vi "OpenConfigFile.vi"(8 "error in (no error)":errorcluster, 10 "ms timeout (2000)":i32=2000, 11 "configuration file path":path) -> (0 "error out":errorcluster, 2 "timeout":bool, 3 "refnum":T1)   [LabVIEW 2020, in "ViewableActor.lvlib"]
doc: "Opens a reference to the configuration data found in a platform-independent configuration file."
uses:
  <vilib>/Utility/config.llb/Config Data RefNum.ctl
  ViewableActor.lvlib
  <vilib>/Utility/config.llb/NI_LVConfig.lvlib
  <vilib>/Utility/error.llb/DialogType.ctl
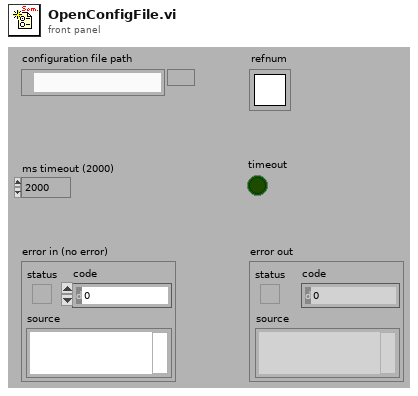
[diagram p1: front panel]
types:
  T1 = typedef "NI_LVConfig.lvlib/Config Data RefNum.ctl" = refnum<k1>
  T2 = typedef "Semaphore RefNum" = refnum<k1>
  T3 = typedef "DialogType.ctl" = u16
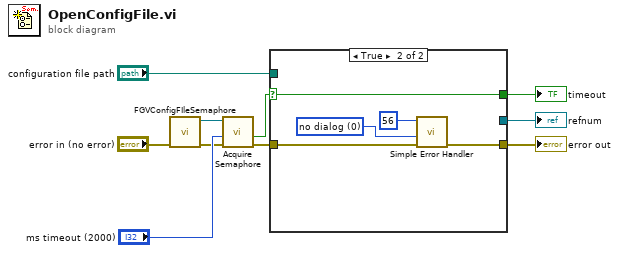
[diagram p0: block diagram]
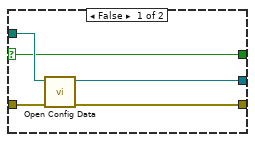
[diagram p2: hidden frame]
diagram:
  n1 = call "FGVConfigFIleSemaphore.vi"("error in (no error)"="error in (no error)") -> ("error out"=w9:errorcluster, "semaphore"=w1:T2)  [unwired: 9 in]
  n2 = call <vilib>:"Acquire Semaphore.vi"("error in (no error)"=w9, "ms timeout (-1)"="ms timeout (2000)", "semaphore"=w1) -> ("error out"=w6:errorcluster, "timed out"=w3:bool)  [unwired: 2 in, 1 out]
  n3 = case shown="True" w3 {
    selector: w3 -> [w11 w19]
    tunnel: "configuration file path" -> [w15 _]
    tunnel: w6 -> [w14 w20]
    tunnel: [w13 _] -> w5
    tunnel: [w12 w18] -> w4
    tunnel: [w11 w19] -> w2
    frame False {
      n4 = call <vilib>:"Open Config Data.vi"("error in (no error)"=w14, "configuration file path"=w15) -> ("error out"=w12:errorcluster, "refnum"=w13:T1)  [unwired: 7 in, 1 out]
    }
    frame True {
      w16 = T3 0 items=["no dialog", "OK message", "continue or stop message", "OK message + warnings", "continue/stop + warnings"] ("type of dialog (OK msg:1)")
      n5 = call <vilib>:"Simple Error Handler.vi"("error code (no error:0)"=56, "type of dialog (OK msg:1)"=w16, "error in (no error)"=w20) -> ("error out"=w18:errorcluster)  [unwired: 2 in, 4 out]
    }
  }
  "error out" <- w4
  "timeout" <- w2
  "refnum" <- w5
